vi "HFRR ADV v11.vi"() -> ()   [LabVIEW 2025] (continued)
                    n421 = Bundle By Name(cluster=w701, "average"=w692) -> (w699:cluster{"major":dbl, "minor":dbl, "average":dbl})
                    n422 = Number To Fractional String(number=w692, precision (6)=i16 1) -> (F-format string=w691:string)  [unwired: 2 in]
                    n423 = local write "Minor Axis"(w697) -> ()
                    n424 = local write "Major Axis"(w697) -> ()
                    n425 = Fract/Exp String To Number(string=w691) -> (number=w690:dbl)  [unwired: 3 in, 1 out]
                    n426 = local write "Average"(w690) -> ()
                  }
                }
              }
              frame True {
                w729 = 1000.0 ("y")
                w735 = 0.0 ("default (0 DBL)")
                n427 = Match Pattern(string=w741, regular expression=" \"width_px\":") -> (after substring=w739:string)  [unwired: 1 in, 3 out]
                n428 = Match Pattern(string=w739, regular expression="\"height_px\":") -> (before substring=w737:string, after substring=w736:string)  [unwired: 1 in, 2 out]
                n429 = Fract/Exp String To Number(string=w737, default (0 dbl)=w735) -> (number=w734:dbl)  [unwired: 2 in, 1 out]
                n430 = Fract/Exp String To Number(string=w736, default (0 dbl)=w735) -> (number=w733:dbl)  [unwired: 2 in, 1 out]
                n431 = Multiply(x=w734, y=w732) -> (x*y=w731:dbl)
                n432 = Multiply(x=w733, y=w732) -> (x*y=w730:dbl)
                n433 = Multiply(x=w731, y=w729) -> (x*y=w715:dbl)
                n434 = Multiply(x=w730, y=w729) -> (x*y=w713:dbl)
                n435 = Add(x=w715, y=w713) -> (x+y=w727:dbl)
                n436 = property on="Major Axis" class="DigNum (strict)"("Caption.Text"="Major Axis") -> ()  [unwired: 2 in, 2 out]
                n437 = property on="Minor Axis" class="DigNum (strict)"("Caption.Text"="Minor Axis") -> ()  [unwired: 2 in, 2 out]
                n438 = property on="Average" class="DigNum (strict)"("Caption.Text"="Average") -> ()  [unwired: 2 in, 2 out]
                n439 = Divide(x=w727, y=2.0) -> (x/y=w711:dbl)
                n440 = Bundle By Name(cluster=w728, "major"=w715, "minor"=w713, "average"=w711) -> (w725:cluster{"major":dbl, "minor":dbl, "average":dbl})
                n441 = Number To Fractional String(number=w713, precision (6)=i16 1) -> (F-format string=w720:string)  [unwired: 2 in]
                n442 = Number To Fractional String(number=w711, precision (6)=i16 1) -> (F-format string=w721:string)  [unwired: 2 in]
                n443 = Number To Fractional String(number=w715, precision (6)=i16 1) -> (F-format string=w719:string)  [unwired: 2 in]
                n444 = Fract/Exp String To Number(string=w720) -> (number=w712:dbl)  [unwired: 3 in, 1 out]
                n445 = Fract/Exp String To Number(string=w721) -> (number=w710:dbl)  [unwired: 3 in, 1 out]
                n446 = Fract/Exp String To Number(string=w719) -> (number=w714:dbl)  [unwired: 3 in, 1 out]
                n447 = local write "Major Axis"(w714) -> ()
                n448 = local write "Average"(w710) -> ()
                n449 = local write "Minor Axis"(w712) -> ()
              }
            }
            n450 = case shown="\"Measrument\", Default" w624 {
              tunnel: w627 -> [w654 _]
              tunnel: w626 -> [w653 _]
              tunnel: [w650 w679] -> w625
              tunnel: w623 -> [w652 w679]
              tunnel: w622 -> [w651 _]
              tunnel: w619 -> [w649 _]
              frame "Measrument", Default {
                n451 = stacked-sequence {
                  tunnel: w654 -> [w672 _]
                  tunnel: w653 -> [w670 _]
                  tunnel: w652 -> [w668 _]
                  tunnel: w651 -> [w667 _]
                  tunnel: [w662 _] -> w650
                  tunnel: w649 -> [w655 _]
                  frame #0 {
                    n452 = call "IMAGE ANALYSIS.vi"("Enum"=POST_ANALYSIS_ENUM."SAVE IMAGE", "error in"=w668, "IMAGE FILE PATH"=w667) -> ("error out"=w666:errorcluster)  [unwired: 7 in, 1 out]
                    n453 = call "Stall Data Flow.vim"("value in"=w666, "milliseconds to wait"=u32 1000) -> ("value out"=w657:errorcluster)  [unwired: 1 out]
                    n454 = local read "Test File List :"() -> (w674:string)
                    n455 = call "IMAGE ANALYSIS.vi"("Enum"=POST_ANALYSIS_ENUM."MINIMIZE UI", "error in"=w657) -> ("error out"=w664:errorcluster)  [unwired: 8 in, 1 out]
                    n456 = Bundle By Name(cluster=T21 {"File Name"="", "Test Method"="", "Operator"="", "Fuel Description"="", "Date and time"=""} ("Main Ref"), "Test Method"=w655, "File Name"=w674) -> (w675:T21)
                    n457 = call "Stall Data Flow.vim"("value in"=w664, "milliseconds to wait"=u32 1500) -> ("value out"=w659:errorcluster)  [unwired: 1 out]
                    n458 = call "duf file read.vi"("error in (no error)"=w659, "Main Ref"=w675) -> ("error out"=w673:errorcluster, "Main Ref 2"=w671:T21)  [unwired: 8 in]
                    n459 = call "DETECTION REPORT for manual.vi"("error in (no error)"=w673, "return value 3"=w670, "Image File Path"=w672, "Main Ref"=w671) -> ("error out"=w669:errorcluster)  [unwired: 7 in]
                    n460 = call <vilib>:"Clear Errors.vi"("error in (no error)"=w669) -> ("error out"=w660:errorcluster)  [unwired: 5 in, 1 out]
                    n461 = call "IMAGE ANALYSIS.vi"("Enum"=POST_ANALYSIS_ENUM."MINIMIZE UI", "error in"=w660) -> ("error out"=w662:errorcluster)  [unwired: 8 in, 1 out]
                  }
                  frame #1 {
                    n462 = local write "Main Tab"(T2."HOME" ("Main Tab")) -> ()
                    n463 = local write "Main Dashboard Buttons"(T1."Home" ("Main Dashboard Buttons")) -> ()
                  }
                }
              }
              frame "Calibrate" {
              }
            }
          }
          frame #2 {
            n464 = Not(x=w744) -> (.not. x?=w743:bool)
            n465 = local write "Confirm Measrurement"(w743) -> ()
            n466 = local read "Calibration Tab"() -> (w742:enum32{"Measrument", "Calibrate"})
            n467 = case shown="\"Measrument\", Default" w742 {
              frame "Measrument", Default {
                n468 = local write "Main Tab"(T2."HOME" ("Main Tab")) -> ()
              }
              frame "Calibrate" {
              }
            }
          }
        }
      }
    }
    n469 = local read "Humidity"() -> (w487:bool)
    n470 = local read "Save Change"() -> (w492:bool)
    n471 = local read "Calibrate"() -> (w493:bool)
    n472 = local read "Auto Start Test"() -> (w488:bool)
    n473 = case shown="True" w493 {
      selector: w493 -> [_ w600]
      frame False {
      }
      frame True {
        n474 = Not(x=w600) -> (.not. x?=w599:bool)
        n475 = local write "Calibrate"(w599) -> ()
        n476 = local write "Calibration Tab"(enum32{"Measrument", "Calibrate"}."Calibrate" ("Calibration Tab")) -> ()
      }
    }
    n477 = case shown="True" w492 {
      selector: w492 -> [_ w544]
      frame False {
      }
      frame True {
        n478 = stacked-sequence {
          tunnel: w544 -> [_ _ _ _ w598]
          frame #0 {
            n479 = call "IMAGE ANALYSIS.vi"("Enum"=POST_ANALYSIS_ENUM."HIDE UI") -> ()  [unwired: 9 in, 2 out]
          }
          frame #1 {
            n480 = local read "100x gain"() -> (w546:dbl)
            n481 = local read "10x Gain"() -> (w547:dbl)
            n482 = local read "5x Gain"() -> (w548:dbl)
            n483 = Number To Fractional String(number=w547, width (-)=i16 4, precision (6)=i16 7) -> (F-format string=w569:string)  [unwired: 1 in]
            n484 = Number To Fractional String(number=0.0, width (-)=i16 4, precision (6)=i16 7) -> (F-format string=w564:string)  [unwired: 1 in]
            n485 = Number To Fractional String(number=w546, width (-)=i16 4, precision (6)=i16 7) -> (F-format string=w552:string)  [unwired: 1 in]
            n486 = Number To Fractional String(number=w548, width (-)=i16 10 ("precision (6)"), precision (6)=i16 7) -> (F-format string=w578:string)  [unwired: 1 in]
            n487 = Concatenate Strings("[CH1]" ("string"), w578, " - 5x Gain" ("string"), "\r") -> (w568:string)
            n488 = Concatenate Strings("[CH2]" ("string"), w569, " - 10x Gain" ("string"), "\r") -> (w567:string)
            n489 = Concatenate Strings("[CH3]" ("string"), w564, " - 20x Gain" ("string"), "\r") -> (w558:string)
            n490 = Concatenate Strings("[CH4]" ("string"), w552, " - 100x Gain" ("string"), "\r") -> (w551:string)
            n491 = String To Path(string="C:\\LAB-IQ\\Image Calibrate v01.dcf") -> (path=w581:path)
            n492 = Concatenate Strings(w568, w567, w558, w551) -> (w566:string)
            n493 = call <vilib>:"Write Characters To File.vi"("append to file? (new file:F)"=FALSE, "character string"=w566, "file path (dialog if empty)"=w581) -> ()  [unwired: 2 in, 1 out]
          }
          frame #2 {
            n494 = String To Path(string="C:\\LAB-IQ\\Image Calibrate v01.dcf") -> (path=w584:path)
            n495 = Open/Create/Replace File ("Open File")(file path (use dialog)=w584) -> (refnum out=w585:refnum<file>)  [unwired: 5 in, 2 out]
            n496 = for {
              N: 4 -> [_]
              tunnel: w585 -> [w591]
              i -> [w587]
              n497 = Read from Text File ("Read File")(file (use dialog)=w591) -> (text=w592:string)  [unwired: 3 in, 3 out]
              n498 = String Subset(string=w592, offset (0)=6, length (rest)=10 ("length (rest)")) -> (substring=w588:string)
              n499 = Fract/Exp String To Number(string=w588) -> (number=w586:dbl)  [unwired: 3 in, 1 out]
              n500 = case shown="3" w587 {
                tunnel: w586 -> [w593 w594 _ w595 _]
                frame 0 {
                  n501 = local write "5x Gain"(w593) -> ()
                }
                frame 1 {
                  n502 = local write "10x Gain"(w594) -> ()
                }
                frame 2 {
                }
                frame 3 {
                  n503 = local write "100x gain"(w595) -> ()
                }
                frame 4, Default {
                }
              }
            }
          }
          frame #3 {
            n504 = call "IMAGE ANALYSIS.vi"("Enum"=POST_ANALYSIS_ENUM."SHOW UI") -> ()  [unwired: 9 in, 2 out]
          }
          frame #4 {
            n505 = Not(x=w598) -> (.not. x?=w597:bool)
            n506 = local write "Save Change"(w597) -> ()
          }
        }
      }
    }
    n507 = case shown="False" w488 {
      tunnel: w487 -> [w514 _]
      frame False {
        n508 = case shown="True" w514 {
          frame False {
          }
          frame True {
            n509 = local read "Set Humidity:"() -> (w518:dbl)
            n510 = local read "Set Humidity:"() -> (w521:dbl)
            n511 = local read "Humidity ( %RH )"() -> (w522:dbl)
            n512 = Subtract(x=w518, y=2.0) -> (x-y=w516:dbl)
            n513 = Add(x=w521, y=2.0) -> (x+y=w517:dbl)
            n514 = In Range and Coerce(upper limit=w517, x=w522, lower limit=w516) -> (In Range?=w515:bool)  [unwired: 1 out]
            n515 = case shown="True" w515 {
              frame False {
              }
              frame True {
                n516 = case shown="False" "Manual Humididty Reached" {
                  selector: "Manual Humididty Reached" -> [_ w525]
                  frame False {
                  }
                  frame True {
                    n517 = Not(x=w525) -> (.not. x?=w524:bool)
                    n518 = local write "Manual Humididty Reached"(w524) -> ()
                    n519 = local read "EVENT LOG"() -> (w527:string)
                    n520 = call "Event Log.vi"("Content"="Target Humidity reached", "EVENT LOG"=w527) -> ("EVENT LOG"=w526:string)  [unwired: 8 in, 1 out]
                    n521 = local write "EVENT LOG"(w526) -> ()
                  }
                }
              }
            }
          }
        }
      }
      frame True {
        n522 = local write "Manual Humididty Reached"(TRUE ("Manual Humididty Reached")) -> ()
      }
    }
    n523 = local read "Cap Live Image"() -> (w508:bool)
    n524 = local read "SCAR MEASURMENT"() -> (w511:enum32{"Auto Scar", "Manual Scar"})
    n525 = Wait (ms)(milliseconds to wait=u32 250) -> ()  [unwired: 1 out]
    n526 = Equal?(x=w511, y=enum32{"Auto Scar", "Manual Scar"}."Manual Scar" ("SCAR MEASURMENT")) -> (x = y?=w509:bool)
    n527 = And(x=w509, y=w508) -> (x .and. y?=w507:bool)
    n528 = case shown="True" w507 {
      selector: w507 -> [_ w823]
      frame False {
      }
      frame True {
        n529 = stacked-sequence {
          tunnel: [_ _ _ w838 _] -> _
          tunnel: w823 -> [_ _ _ _ w844]
          frame #0 {
            w824 = 0.0
            n530 = local write "Major Axis"(w824) -> ()
            n531 = local write "Minor Axis"(w824) -> ()
            n532 = local write "Average"(w824) -> ()
          }
          frame #1 {
            n533 = call "CAMERA LIVE FEED FGV.vi"("Enum - Menu"=CAMERA_LIVE_FEED_ENUM."CAMERA MINIMIZE") -> ()  [unwired: 9 in, 2 out]
          }
          frame #2 {
            n534 = local read "FILE 3"() -> (w832:string)
            n535 = call <vilib>:"Trim Whitespace.vi"("string"="C:\\LAB-IQ\\images\\") -> ("trimmed string"=w834:string)  [unwired: 1 in]
            n536 = String To Path(string=w834) -> (path=w833:path)
            n537 = Concatenate Strings(w832, ".png" ("string")) -> (w831:string)
            n538 = Build Path(base path=w833, name or relative path=w831) -> (appended path=w829:path)
            n539 = Path To String(path=w829) -> (string=w828:string)
            n540 = call "CAMERA LIVE FEED FGV.vi"("Enum - Menu"=CAMERA_LIVE_FEED_ENUM."CAMERA SAVE", "Image Path"=w828) -> ("error out"=w826:errorcluster)  [unwired: 8 in, 1 out]
            n541 = case shown="No Error" w826 {
              frame No Error {
                n542 = One Button Dialog(message="Image saved successfully") -> ()  [unwired: 1 in, 1 out]
              }
              frame Error {
              }
            }
          }
          frame #3 {
            n543 = call "LIST FILE NAMES.vi"() -> ("error out"=w840:errorcluster, "filenames"=w837:string[])  [unwired: 10 in]
            n544 = call "IMAGE ANALYSIS.vi"("Enum"=POST_ANALYSIS_ENUM."SHOW UI", "error in"=w840) -> ("error out"=w838:errorcluster)  [unwired: 8 in, 1 out]
            n545 = property on="Test File List :" class="CmbBox"("Strings[]"=w837) -> ()  [unwired: 2 in, 2 out]
          }
          frame #4 {
            (unwired) T22."Report" ("Main Dashboard Buttons")
            n546 = Not(x=w844) -> (.not. x?=w843:bool)
            n547 = local write "Zoom Factore"(0.0 ("Zoom Factore")) -> ()
            n548 = local write "Cap Live Image"(w843) -> ()
            n549 = local write "Main Tab"(T2."Adv Scar Report" ("Main Tab")) -> ()
            n550 = property on="Cap Live Image" class="Bool (strict)"("BoolText.Text"="Capture Image" ("Boolean Text.Text")) -> ()  [unwired: 2 in, 2 out]
            n551 = local write "Main Dashboard Buttons"(T1."Report" ("Main Dashboard Buttons")) -> ()
          }
        }
      }
    }
    n552 = local read "change Gain"() -> (w491:bool)
    n553 = local read "Back Square"() -> (w490:bool)
    n554 = case shown="True" w491 {
      selector: w491 -> [_ w535]
      frame False {
      }
      frame True {
        n555 = stacked-sequence {
          tunnel: w535 -> [_ w543]
          frame #0 {
            n556 = local read "Actual (µm)"() -> (w539:dbl)
            n557 = local read "Pixel Value"() -> (w538:dbl)
            n558 = local read "Magnification :"() -> (w537:string)
            n559 = Divide(x=w539, y=w538) -> (x/y=w536:dbl)
            n560 = case shown="\"10x\"" w537 {
              tunnel: w536 -> [w540 w541]
              frame "10x" {
                n561 = local write "10x Gain"(w540) -> ()
              }
              frame "5x", Default {
                n562 = local write "5x Gain"(w541) -> ()
              }
            }
          }
          frame #1 {
            n563 = Not(x=w543) -> (.not. x?=w542:bool)
            n564 = local write "change Gain"(w542) -> ()
          }
        }
      }
    }
    n565 = case shown="True" w490 {
      selector: w490 -> [_ w533]
      frame False {
      }
      frame True {
        n566 = Not(x=w533) -> (.not. x?=w532:bool)
        n567 = local write "Back Square"(w532) -> ()
        n568 = local write "Calibration Tab"(enum32{"Measrument", "Calibrate"}."Measrument" ("Calibration Tab")) -> ()
      }
    }
    n569 = local read "Rectangle Tool"() -> (w502:bool)
    n570 = local read "Clear ROI Tool"() -> (w501:bool)
    n571 = local read "Open Image"() -> (w506:bool)
    n572 = local read "line tool"() -> (w503:bool)
    n573 = local read "OUT"() -> (w504:bool)
    n574 = local read "In"() -> (w505:bool)
    n575 = case shown="True" w506 {
      selector: w506 -> [_ w811]
      tunnel: [w807 w813] -> _
      tunnel: w496 -> [w807 w812]
      frame False {
      }
      frame True {
        n576 = Not(x=w811) -> (.not. x?=w810:bool)
        n577 = local write "Open Image"(w810) -> ()
        n578 = call "IMAGE ANALYSIS.vi"("Enum"=POST_ANALYSIS_ENUM."HIDE UI", "error in"=w812) -> ("error out"=w820:errorcluster)  [unwired: 8 in, 1 out]
        n579 = call "File Dialog"("start path"=path "C:/LAB-IQ/images", "error in"=w820) -> ("selected path"=w809:path, "error out"=w818:errorcluster)  [unwired: 10 in, 2 out]
        "Image path  2" <- w809
        n580 = call <vilib>:"Clear Errors.vi"("error in (no error)"=w818) -> ("error out"=w817:errorcluster)  [unwired: 5 in, 1 out]
        n581 = call "IMAGE ANALYSIS.vi"("Enum"=POST_ANALYSIS_ENUM."OPEN FILE", "error in"=w817, "File Path"=w809) -> ("error out"=w816:errorcluster)  [unwired: 7 in, 1 out]
        n582 = call <vilib>:"Clear Errors.vi"("error in (no error)"=w816) -> ("error out"=w815:errorcluster)  [unwired: 5 in, 1 out]
        n583 = call "IMAGE ANALYSIS.vi"("Enum"=POST_ANALYSIS_ENUM."SHOW UI", "error in"=w815) -> ("error out"=w813:errorcluster)  [unwired: 8 in, 1 out]
        n584 = local write "Zoom Factore"(100.0 ("Zoom Factore")) -> ()
      }
    }
    n585 = case shown="True" w504 {
      selector: w504 -> [_ w792]
      tunnel: w496 -> [w789 w797]
      tunnel: [w789 w791] -> _
      frame False {
      }
      frame True {
        n586 = Not(x=w792) -> (.not. x?=w790:bool)
        n587 = local read "Zoom Factore"() -> (w795:dbl)
        n588 = local write "OUT"(w790) -> ()
        n589 = call "IMAGE ANALYSIS.vi"("Enum"=POST_ANALYSIS_ENUM."ZOOM OUT", "error in"=w797) -> ("error out"=w791:errorcluster)  [unwired: 8 in, 1 out]
        n590 = Divide(x=w795, y=1.2) -> (x/y=w793:dbl)
        n591 = local write "Zoom Factore"(w793) -> ()
      }
    }
    n592 = case shown="True" w505 {
      selector: w505 -> [_ w801]
      tunnel: w496 -> [w798 w806]
      tunnel: [w798 w799] -> _
      frame False {
      }
      frame True {
        n593 = Not(x=w801) -> (.not. x?=w800:bool)
        n594 = local read "Zoom Factore"() -> (w804:dbl)
        n595 = local write "In"(w800) -> ()
        n596 = call "IMAGE ANALYSIS.vi"("Enum"=POST_ANALYSIS_ENUM."ZOOM IN", "error in"=w806) -> ("error out"=w799:errorcluster)  [unwired: 8 in, 1 out]
        n597 = Multiply(x=w804, y=1.2) -> (x*y=w802:dbl)
        n598 = local write "Zoom Factore"(w802) -> ()
      }
    }
    n599 = case shown="True" w501 {
      selector: w501 -> [_ w773]
      tunnel: w496 -> [w771 w775]
      tunnel: [w771 w774] -> _
      frame False {
      }
      frame True {
        n600 = Not(x=w773) -> (.not. x?=w772:bool)
        n601 = local write "Clear ROI Tool"(w772) -> ()
        n602 = call "IMAGE ANALYSIS.vi"("Enum"=POST_ANALYSIS_ENUM."CLEAR ROI", "error in"=w775) -> ("error out"=w774:errorcluster)  [unwired: 8 in, 1 out]
      }
    }
    n603 = case shown="True" w503 {
      selector: w503 -> [_ w785]
      tunnel: w496 -> [w783 w788]
      tunnel: [w783 w786] -> _
      frame False {
      }
      frame True {
        n604 = Not(x=w785) -> (.not. x?=w784:bool)
        n605 = local write "line tool"(w784) -> ()
        n606 = call "IMAGE ANALYSIS.vi"("Enum"=POST_ANALYSIS_ENUM."DRAW LINE", "error in"=w788) -> ("error out"=w786:errorcluster)  [unwired: 8 in, 1 out]
      }
    }
    n607 = case shown="True" w502 {
      selector: w502 -> [_ w779]
      tunnel: w496 -> [w777 w781]
      tunnel: [w777 w780] -> _
      frame False {
      }
      frame True {
        n608 = Not(x=w779) -> (.not. x?=w778:bool)
        n609 = local write "Rectangle Tool"(w778) -> ()
        n610 = call "IMAGE ANALYSIS.vi"("Enum"=POST_ANALYSIS_ENUM."DRAW REC", "error in"=w781) -> ("error out"=w780:errorcluster)  [unwired: 8 in, 1 out]
      }
    }
    n611 = local read "SCAR MEASURMENT"() -> (w489:enum32{"Auto Scar", "Manual Scar"})
    n612 = local read "Fit to Screen Tool"() -> (w498:bool)
    n613 = local read "Resize Tool"() -> (w497:bool)
    n614 = case shown="\"Manual Scar\", Default" w489 {
      frame "Auto Scar" {
        n615 = property on="Cap Live Image" class="Bool (strict)"("BoolText.Text"="Report" ("Boolean Text.Text")) -> ()  [unwired: 2 in, 2 out]
      }
      frame "Manual Scar", Default {
        n616 = property on="Cap Live Image" class="Bool (strict)"("BoolText.Text"="Save Image" ("Boolean Text.Text")) -> ()  [unwired: 2 in, 2 out]
      }
    }
    n617 = local read "ROI Color Tool"() -> (w499:bool)
    n618 = local read "Pan Tool"() -> (w500:bool)
    n619 = case shown="True" w500 {
      selector: w500 -> [_ w767]
      tunnel: w496 -> [w765 w769]
      tunnel: [w765 w768] -> _
      frame False {
      }
      frame True {
        n620 = Not(x=w767) -> (.not. x?=w766:bool)
        n621 = call "IMAGE ANALYSIS.vi"("Enum"=POST_ANALYSIS_ENUM."PAN", "error in"=w769) -> ("error out"=w768:errorcluster)  [unwired: 8 in, 1 out]
        n622 = local write "Pan Tool"(w766) -> ()
      }
    }
    n623 = case shown="True" w497 {
      selector: w497 -> [_ w751]
      tunnel: w496 -> [w746 w748]
      tunnel: [w746 w747] -> _
      frame False {
      }
      frame True {
        n624 = Not(x=w751) -> (.not. x?=w750:bool)
        n625 = local write "Resize Tool"(w750) -> ()
        n626 = call "IMAGE ANALYSIS.vi"("Enum"=POST_ANALYSIS_ENUM."RESIZE MODE", "error in"=w748) -> ("error out"=w747:errorcluster)  [unwired: 8 in, 1 out]
      }
    }
    n627 = case shown="True" w498 {
      selector: w498 -> [_ w756]
      tunnel: [w752 w757] -> _
      tunnel: w496 -> [w752 w755]
      frame False {
      }
      frame True {
        n628 = Not(x=w756) -> (.not. x?=w754:bool)
        n629 = local write "Zoom Factore"(100.0 ("Zoom Factore")) -> ()
        n630 = local write "Fit to Screen Tool"(w754) -> ()
        n631 = call "IMAGE ANALYSIS.vi"("Enum"=POST_ANALYSIS_ENUM."FIT", "error in"=w755) -> ("error out"=w757:errorcluster)  [unwired: 8 in, 1 out]
      }
    }
    n632 = case shown="True" w499 {
      selector: w499 -> [_ w762]
      tunnel: [w759 w763] -> _
      tunnel: w496 -> [w759 w760]
      frame False {
      }
      frame True {
        n633 = Not(x=w762) -> (.not. x?=w761:bool)
        n634 = local write "ROI Color Tool"(w761) -> ()
        n635 = call "IMAGE ANALYSIS.vi"("Enum"=POST_ANALYSIS_ENUM."SET ROI COLOR", "error in"=w760) -> ("error out"=w763:errorcluster)  [unwired: 8 in, 1 out]
      }
    }
    n636 = local read "Quit"() -> (w513:bool)
  }
  n637 = local write "USERNAME"(w28) -> ()
  n638 = local write "Main Tab"(T2."HOME" ("Main Tab")) -> ()
  n639 = local write "USER ID"(w28) -> ()
  n640 = property on="Auto Scar Check  2" class="Clust (strict)"("Visible"=w9) -> (error out=w13:errorcluster)  [unwired: 2 in, 1 out]
  n641 = property on="Quit" class="Bool (strict)"("Value"=FALSE ("Quit")) -> (error out=w30:errorcluster)  [unwired: 2 in, 1 out]
  n642 = while {
    stop <- w847 stop-if-true
    n643 = local read "Image Path"() -> (w850:path)
    n644 = local read "Print 3"() -> (w853:bool)
    n645 = Equal?(x=w850, y=path "") -> (x = y?=w849:bool)
    n646 = Not(x=w849) -> (.not. x?=w848:bool)
    n647 = property on="Print 3" class="Bool (strict)"("Visible"=w848) -> ()  [unwired: 2 in, 2 out]
    n648 = case shown="True" w853 {
      frame False {
        n649 = local write "Rd"(TRUE ("Boolean 7")) -> ()
      }
      frame True {
        n650 = flat-sequence {
          tunnel: [w893] -> w861
          tunnel: [w880] -> w859
          tunnel: [w890] -> w855
          tunnel: w861 -> [w902]
          tunnel: [w902] -> w860
          tunnel: w859 -> [w901]
          tunnel: [w901] -> w858
          tunnel: [w899] -> w857
          tunnel: [w898] -> w856
          tunnel: w855 -> [w898]
          tunnel: w860 -> [w904]
          tunnel: w858 -> [w905]
          tunnel: w857 -> [_]
          tunnel: w856 -> [w903]
          frame #0 {
            n651 = case shown="True" "Rd" {
              frame False {
              }
              frame True {
                n652 = while {
                  tunnel: "abcdefABCDEF" ("string 2") -> [w872]
                  shift-right: [w870] -> w864
                  shift-left: "" -> [w869]
                  i -> [w879]
                  stop <- w878 stop-if-true
                  n653 = Random Number (0-1)() -> (number: 0 to 1=w873:dbl)
                  n654 = Multiply(x=w873, y=62.0) -> (x*y=w875:dbl)
                  n655 = Decrement(x="Length 2") -> (x-1=w868:i16)
                  n656 = To Word Integer(number=w875) -> (16bit integer=w876:i16)
                  n657 = String Subset(string=w872, offset (0)=w876, length (rest)=1 ("length (rest)")) -> (substring=w871:string)
                  n658 = Greater Or Equal?(x=w879, y=w868) -> (x >= y?=w878:bool)
                  n659 = Concatenate Strings(w871, w869) -> (w870:string)
                }
                "String 10" <- w864
                n660 = local write "Rd"(FALSE ("Boolean 7")) -> ()
              }
            }
          }
          frame #1 {
            w891 = "_resized.jpg" ("command line")
            (unwired) ".jpg -resize 320x240 " ("string")
            (unwired) "Choose an Image File" ("prompt")
            # "-resize 1798x425"
            n661 = local read "Image Path"() -> (w885:path)
            n662 = Strip Path(path=w885) -> (stripped path=w880:path, name=w881:string)
            n663 = Match Pattern(string=w881, regular expression=".jpg") -> (before substring=→"before substring 2":string, after substring=→"after substring":string)  [unwired: 1 in, 2 out]
            n664 = Match Pattern(string=w881, regular expression="\\") -> (before substring=w887:string)  [unwired: 1 in, 3 out]
            n665 = Match Pattern(string=w887, regular expression=".jpg") -> (before substring=w886:string)  [unwired: 1 in, 3 out]
            n666 = Concatenate Strings("cmd /c convert " ("string"), w886, ".jpg -resize 320x240  " ("command line"), w886, w891) -> (w894:string)
            n667 = call <vilib>:"System Exec.vi"("run minimized? (F)"=TRUE, "wait until completion? (T)"=TRUE, "working directory"=w880, "command line"=w894) -> ("error out"=w893:errorcluster)  [unwired: 4 in, 3 out]
            "error out 2" <- w893
            n668 = Concatenate Strings(w886, w891) -> (w890:string)
          }
          frame #2 {
            n669 = Wait (ms)(milliseconds to wait=u32 2000 ("millisecond timer value")) -> (millisecond timer value=w899:u32)
          }
          frame #3 {
            n670 = case shown="No Error" w904 {
              tunnel: w905 -> [w908 _]
              tunnel: w903 -> [w906 _]
              frame No Error {
                (unwired) ".jpg" ("string")
                n671 = Path To String(path=w908) -> (string=w912:string)
                n672 = Concatenate Strings(w912, "\\" ("string"), w906) -> (w911:string)
                n673 = String To Path(string=w911) -> (path=w910:path)
                n674 = call <vilib>:"Read JPEG File.vi"("path to JPEG file"=w910) -> ("image data"=w914:T14)  [unwired: 8 in, 2 out]
                "image data" <- w914
                n675 = local write "Print 3"(FALSE ("Print 2")) -> ()
                n676 = call <vilib>:"Draw Flattened Pixmap.vi"("image data"=w914) -> ("new picture"=→"new picture":picture)  [unwired: 8 in]
              }
              frame Error {
              }
            }
          }
        }
      }
    }
    n677 = Wait (ms)(milliseconds to wait=u32 20 ("millisecond timer value")) -> ()  [unwired: 1 out]
    n678 = local read "Quit"() -> (w847:bool)
  }
  n679 = property on="Service Password Log" class="Str"("Visible"=w9) -> ()  [unwired: 2 in, 2 out]
  n680 = property on="Password 3" class="Clust (strict)"("Visible"=w9) -> ()  [unwired: 2 in, 2 out]
  n681 = while {
    tunnel: w30 -> [_]
    tunnel: w13 -> [_]
    stop <- w945 stop-if-true
    # "New Adv Logics"
    n682 = local read "Main Tab"() -> (w943:T2)
    n683 = local read "Sign In"() -> (w942:bool)
    n684 = local read "Main Tab"() -> (w924:T2)
    n685 = case shown="\"Mooha\"" w924 {
      frame "HOME", Default {
        n686 = local read "LIVE FEED MIN TEMP"() -> (w1072:bool)
        n687 = local write "LIVE FEED MAX TEMP"(TRUE ("LIVE FEED MAX TEMP")) -> ()
        n688 = local read "CAMERA ROI MIN TEMP"() -> (w1070:bool)
        n689 = case shown="True" w1072 {
          selector: w1072 -> [_ w1079]
          frame False {
          }
          frame True {
            n690 = Not(x=w1079) -> (.not. x?=w1078:bool)
            n691 = local write "LIVE FEED MIN TEMP"(w1078) -> ()
            n692 = call "CAMERA LIVE FEED FGV.vi"("Enum - Menu"=CAMERA_LIVE_FEED_ENUM."CAMERA MINIMIZE") -> ()  [unwired: 9 in, 2 out]
          }
        }
        n693 = case shown="True" w1070 {
          selector: w1070 -> [_ w1076]
          frame False {
          }
          frame True {
            n694 = Not(x=w1076) -> (.not. x?=w1075:bool)
            n695 = local write "CAMERA ROI MIN TEMP"(w1075) -> ()
            n696 = call "IMAGE ANALYSIS.vi"("Enum"=POST_ANALYSIS_ENUM."MINIMIZE UI") -> ()  [unwired: 9 in, 2 out]
          }
        }
        n697 = local write "CAMERA ROI MAX TEMP"(TRUE ("CAMERA ROI MAX TEMP")) -> ()
      }
      frame "Test Setup" {
        n698 = local read "LIVE FEED MIN TEMP"() -> (w1082:bool)
        n699 = local read "CAMERA ROI MIN TEMP"() -> (w1080:bool)
        n700 = local write "LIVE FEED MAX TEMP"(TRUE ("LIVE FEED MAX TEMP")) -> ()
        n701 = case shown="True" w1082 {
          selector: w1082 -> [_ w1089]
          frame False {
          }
          frame True {
            n702 = Not(x=w1089) -> (.not. x?=w1088:bool)
            n703 = local write "LIVE FEED MIN TEMP"(w1088) -> ()
            n704 = call "CAMERA LIVE FEED FGV.vi"("Enum - Menu"=CAMERA_LIVE_FEED_ENUM."CAMERA MINIMIZE") -> ()  [unwired: 9 in, 2 out]
          }
        }
        n705 = case shown="True" w1080 {
          selector: w1080 -> [_ w1086]
          frame False {
          }
          frame True {
            n706 = Not(x=w1086) -> (.not. x?=w1085:bool)
            n707 = local write "CAMERA ROI MIN TEMP"(w1085) -> ()
            n708 = call "IMAGE ANALYSIS.vi"("Enum"=POST_ANALYSIS_ENUM."MINIMIZE UI") -> ()  [unwired: 9 in, 2 out]
          }
        }
        n709 = local write "CAMERA ROI MAX TEMP"(TRUE ("CAMERA ROI MAX TEMP")) -> ()
      }
      frame "Acquire" {
        n710 = local read "LIVE FEED MIN TEMP"() -> (w1092:bool)
        n711 = local write "LIVE FEED MAX TEMP"(TRUE ("LIVE FEED MAX TEMP")) -> ()
        n712 = local read "CAMERA ROI MIN TEMP"() -> (w1090:bool)
        n713 = case shown="True" w1092 {
          selector: w1092 -> [_ w1099]
          frame False {
          }
          frame True {
            n714 = Not(x=w1099) -> (.not. x?=w1098:bool)
            n715 = local write "LIVE FEED MIN TEMP"(w1098) -> ()
            n716 = call "CAMERA LIVE FEED FGV.vi"("Enum - Menu"=CAMERA_LIVE_FEED_ENUM."CAMERA MINIMIZE") -> ()  [unwired: 9 in, 2 out]
          }
        }
        n717 = case shown="True" w1090 {
          selector: w1090 -> [_ w1096]
          frame False {
          }
          frame True {
            n718 = Not(x=w1096) -> (.not. x?=w1095:bool)
            n719 = local write "CAMERA ROI MIN TEMP"(w1095) -> ()
            n720 = call "IMAGE ANALYSIS.vi"("Enum"=POST_ANALYSIS_ENUM."MINIMIZE UI") -> ()  [unwired: 9 in, 2 out]
          }
        }
        n721 = local write "CAMERA ROI MAX TEMP"(TRUE ("CAMERA ROI MAX TEMP")) -> ()
      }
      frame "Adv Scar" {
        n722 = local read "CAMERA ROI MIN TEMP"() -> (w1100:bool)
        n723 = case shown="True" "LIVE FEED MAX TEMP" {
          selector: "LIVE FEED MAX TEMP" -> [_ w1119]
          frame False {
          }
          frame True {
            n724 = Not(x=w1119) -> (.not. x?=w1118:bool)
            n725 = local write "LIVE FEED MAX TEMP"(w1118) -> ()
            n726 = call "CAMERA LIVE FEED FGV.vi"("Enum - Menu"=CAMERA_LIVE_FEED_ENUM."CAMERA RESTORE") -> ("error out"=w1109:errorcluster)  [unwired: 9 in, 1 out]
            n727 = Type Cast(type=30, x=0) -> (*(type *) &x=w1113:i32)
            n728 = Add(x=w1113, y=48) -> (x+y=w1114:i32)
            n729 = call "CAMERA LIVE FEED FGV.vi"("Enum - Menu"=CAMERA_LIVE_FEED_ENUM."CAMERA MODE SET", "error in (no error)"=w1109, "CAMERA MODE"=w1114) -> ("error out"=w1107:errorcluster)  [unwired: 7 in, 1 out]
            n730 = call "LIST FILE NAMES.vi"("error in (no error)"=w1107) -> ("error out"=w1115:errorcluster, "filenames"=w1116:string[])  [unwired: 9 in]
            n731 = property on="FILE 3" class="CmbBox"(error in=w1115, "Strings[]"=w1116) -> ()  [unwired: 1 in, 2 out]
          }
        }
        n732 = case shown="True" w1100 {
          selector: w1100 -> [_ w1106]
          frame False {
          }
          frame True {
            n733 = Not(x=w1106) -> (.not. x?=w1105:bool)
            n734 = local write "CAMERA ROI MIN TEMP"(w1105) -> ()
            n735 = call "IMAGE ANALYSIS.vi"("Enum"=POST_ANALYSIS_ENUM."MINIMIZE UI") -> ()  [unwired: 9 in, 2 out]
          }
        }
        n736 = local write "CAMERA ROI MAX TEMP"(TRUE ("CAMERA ROI MAX TEMP")) -> ()
        "LIVE FEED MIN TEMP" <- TRUE ("LIVE FEED MIN TEMP")
      }
      frame "Adv Scar Report" {
        n737 = local read "CAMERA ROI MAX TEMP"() -> (w1120:bool)
        n738 = local read "LIVE FEED MIN TEMP"() -> (w1122:bool)
        n739 = local write "LIVE FEED MAX TEMP"(TRUE ("LIVE FEED MAX TEMP")) -> ()
        n740 = case shown="True" w1122 {
          selector: w1122 -> [_ w1131]
          frame False {
          }
          frame True {
            n741 = Not(x=w1131) -> (.not. x?=w1130:bool)
            n742 = local write "LIVE FEED MIN TEMP"(w1130) -> ()
            n743 = call "CAMERA LIVE FEED FGV.vi"("Enum - Menu"=CAMERA_LIVE_FEED_ENUM."CAMERA MINIMIZE") -> ()  [unwired: 9 in, 2 out]
          }
        }
        n744 = case shown="True" w1120 {
          selector: w1120 -> [_ w1128]
          frame False {
          }
          frame True {
            n745 = Not(x=w1128) -> (.not. x?=w1126:bool)
            n746 = local write "CAMERA ROI MAX TEMP"(w1126) -> ()
            n747 = call "IMAGE ANALYSIS.vi"("Enum"=POST_ANALYSIS_ENUM."SHOW UI") -> ("error out"=w1125:errorcluster)  [unwired: 9 in, 1 out]
            n748 = call "LIST FILE NAMES.vi"("error in (no error)"=w1125) -> ("filenames"=w1124:string[])  [unwired: 9 in, 1 out]
            n749 = property on="Test File List :" class="CmbBox"("Strings[]"=w1124) -> ()  [unwired: 2 in, 2 out]
          }
        }
        n750 = local write "CAMERA ROI MIN TEMP"(TRUE ("CAMERA ROI MIN TEMP")) -> ()
      }
      frame "Compare Files" {
        n751 = local read "LIVE FEED MIN TEMP"() -> (w1134:bool)
        n752 = local write "LIVE FEED MAX TEMP"(TRUE ("LIVE FEED MAX TEMP")) -> ()
        n753 = local read "CAMERA ROI MIN TEMP"() -> (w1132:bool)
        n754 = case shown="True" w1134 {
          selector: w1134 -> [_ w1141]
          frame False {
          }
          frame True {
            n755 = Not(x=w1141) -> (.not. x?=w1140:bool)
            n756 = local write "LIVE FEED MIN TEMP"(w1140) -> ()
            n757 = call "CAMERA LIVE FEED FGV.vi"("Enum - Menu"=CAMERA_LIVE_FEED_ENUM."CAMERA MINIMIZE") -> ()  [unwired: 9 in, 2 out]
          }
        }
        n758 = case shown="True" w1132 {
          selector: w1132 -> [_ w1138]
          frame False {
          }
          frame True {
            n759 = Not(x=w1138) -> (.not. x?=w1137:bool)
            n760 = local write "CAMERA ROI MIN TEMP"(w1137) -> ()
            n761 = call "IMAGE ANALYSIS.vi"("Enum"=POST_ANALYSIS_ENUM."MINIMIZE UI") -> ()  [unwired: 9 in, 2 out]
          }
        }
        n762 = local write "CAMERA ROI MAX TEMP"(TRUE ("CAMERA ROI MAX TEMP")) -> ()
      }
      frame "About" {
        n763 = local read "LIVE FEED MIN TEMP"() -> (w1144:bool)
        n764 = local write "LIVE FEED MAX TEMP"(TRUE ("LIVE FEED MAX TEMP")) -> ()
        n765 = local read "CAMERA ROI MIN TEMP"() -> (w1143:bool)
        n766 = case shown="True" w1144 {
          selector: w1144 -> [_ w1151]
          frame False {
          }
          frame True {
            n767 = Not(x=w1151) -> (.not. x?=w1150:bool)
            n768 = local write "LIVE FEED MIN TEMP"(w1150) -> ()
            n769 = call "CAMERA LIVE FEED FGV.vi"("Enum - Menu"=CAMERA_LIVE_FEED_ENUM."CAMERA MINIMIZE") -> ()  [unwired: 9 in, 2 out]
          }
        }
        n770 = case shown="True" w1143 {
          selector: w1143 -> [_ w1148]
          frame False {
          }
          frame True {
            n771 = Not(x=w1148) -> (.not. x?=w1147:bool)
            n772 = local write "CAMERA ROI MIN TEMP"(w1147) -> ()
            n773 = call "IMAGE ANALYSIS.vi"("Enum"=POST_ANALYSIS_ENUM."MINIMIZE UI") -> ()  [unwired: 9 in, 2 out]
          }
        }
        n774 = local write "CAMERA ROI MAX TEMP"(TRUE ("CAMERA ROI MIN TEMP")) -> ()
      }
      frame "Advance" {
        n775 = local read "LIVE FEED MIN TEMP"() -> (w1154:bool)
        n776 = local write "LIVE FEED MAX TEMP"(TRUE ("LIVE FEED MAX TEMP")) -> ()
        n777 = local read "CAMERA ROI MIN TEMP"() -> (w1152:bool)
        n778 = case shown="True" w1154 {
          selector: w1154 -> [_ w1161]
          frame False {
          }
          frame True {
            n779 = Not(x=w1161) -> (.not. x?=w1160:bool)
            n780 = local write "LIVE FEED MIN TEMP"(w1160) -> ()
            n781 = call "CAMERA LIVE FEED FGV.vi"("Enum - Menu"=CAMERA_LIVE_FEED_ENUM."CAMERA MINIMIZE") -> ()  [unwired: 9 in, 2 out]
          }
        }
        n782 = local write "CAMERA ROI MAX TEMP"(TRUE ("CAMERA ROI MAX TEMP")) -> ()
        n783 = case shown="True" w1152 {
          selector: w1152 -> [_ w1158]
          frame False {
          }
          frame True {
            n784 = Not(x=w1158) -> (.not. x?=w1157:bool)
            n785 = local write "CAMERA ROI MIN TEMP"(w1157) -> ()
            n786 = call "IMAGE ANALYSIS.vi"("Enum"=POST_ANALYSIS_ENUM."MINIMIZE UI") -> ()  [unwired: 9 in, 2 out]
          }
        }
      }
      frame "Mooha" {
        n787 = local read "LIVE FEED MIN TEMP"() -> (w1164:bool)
        n788 = local write "LIVE FEED MAX TEMP"(TRUE ("LIVE FEED MAX TEMP")) -> ()
        n789 = local read "CAMERA ROI MIN TEMP"() -> (w1162:bool)
        n790 = case shown="True" w1164 {
          selector: w1164 -> [_ w1171]
          frame False {
          }
          frame True {
            n791 = Not(x=w1171) -> (.not. x?=w1170:bool)
            n792 = local write "LIVE FEED MIN TEMP"(w1170) -> ()
            n793 = call "CAMERA LIVE FEED FGV.vi"("Enum - Menu"=CAMERA_LIVE_FEED_ENUM."CAMERA MINIMIZE") -> ()  [unwired: 9 in, 2 out]
          }
        }
        n794 = local write "CAMERA ROI MAX TEMP"(TRUE ("CAMERA ROI MAX TEMP")) -> ()
        n795 = case shown="True" w1162 {
          selector: w1162 -> [_ w1168]
          frame False {
          }
          frame True {
            n796 = Not(x=w1168) -> (.not. x?=w1167:bool)
            n797 = local write "CAMERA ROI MIN TEMP"(w1167) -> ()
            n798 = call "IMAGE ANALYSIS.vi"("Enum"=POST_ANALYSIS_ENUM."MINIMIZE UI") -> ()  [unwired: 9 in, 2 out]
          }
        }
      }
    }
    n799 = local read "Auto Start Test"() -> (w915:bool)
    n800 = case shown="True" "sign in temp" {
      frame False {
      }
      frame True {
        w952 = 1 ("y")
        n801 = local read "USERNAME"() -> (w958:string)
        n802 = local read "USER ID"() -> (w955:string)
        n803 = call <vilib>:"Trim Whitespace.vi"("string"=w958) -> ("trimmed string"=w957:string)  [unwired: 1 in]
        n804 = call <vilib>:"Trim Whitespace.vi"("string"=w955) -> ("trimmed string"=w956:string)  [unwired: 1 in]
        n805 = String Length(string=w957) -> (length=w954:i32)
        n806 = String Length(string=w956) -> (length=w953:i32)
        n807 = Greater?(x=w954, y=w952) -> (0:w951:bool)
        n808 = Greater?(x=w953, y=w952) -> (0:w950:bool)
        n809 = And(x=w951, y=w950) -> (x .and. y?=w949:bool)
        n810 = case shown="True" w949 {
          frame False {
            n811 = property on="Sign In" class="Bool (strict)"("DisabledEnum"=T16."Disabled" ("Disabled")) -> ()  [unwired: 2 in, 2 out]
          }
          frame True {
            n812 = property on="Sign In" class="Bool (strict)"("DisabledEnum"=T16."Enabled" ("Disabled")) -> ()  [unwired: 2 in, 2 out]
          }
        }
      }
    }
    n813 = local read "Air Temperature"() -> (w932:bool)
    n814 = local read "Coefficient Of Friction"() -> (w933:bool)
    n815 = case shown="False" w915 {
      frame False {
        n816 = local read "Auto stop temp"() -> (w946:bool)
        n817 = case shown="True" w946 {
          frame False {
          }
          frame True {
            n818 = local write "Auto Start Temp"(FALSE ("Auto Start Temp")) -> ()
          }
        }
      }
      frame True {
        "Auto stop temp" <- TRUE ("Auto stop temp")
      }
    }
    n819 = local read "Humidity"() -> (w931:bool)
    n820 = case shown="\"HOME\"" w943 {
      frame "HOME" {
        n821 = local write "main tab sub"(enum32{"Page 1", "Page 2"}."Page 1" ("main tab sub")) -> ()
      }
      frame Default {
        n822 = local write "main tab sub"(enum32{"Page 1", "Page 2"}."Page 2" ("main tab sub")) -> ()
      }
    }
    n823 = case shown="True" w942 {
      selector: w942 -> [_ w1276]
      frame False {
      }
      frame True {
        n824 = Not(x=w1276) -> (.not. x?=w1275:bool)
        n825 = local write "Sign In"(w1275) -> ()
        n826 = local write "Main Dashboard Buttons"(T1."Test Setup" ("Main Dashboard Buttons")) -> ()
      }
    }
    n827 = case shown="\"Numeric Display\", Default" "Num/Graph" {
      frame "Numeric Display", Default {
        n828 = property on="Single/Multiple" class="RadioBtnsControl (strict)"("Visible"=FALSE) -> ()  [unwired: 2 in, 2 out]
        n829 = property on="Single - Graph" class="Ring (strict)"("Visible"=FALSE) -> ()  [unwired: 2 in, 2 out]
        n830 = local write "Main Tab Display"(T4."Dashboard 1" ("Main Tab Display")) -> ()
      }
      frame "Graph Display" {
        n831 = property on="Single/Multiple" class="RadioBtnsControl (strict)"("Visible"=TRUE) -> ()  [unwired: 2 in, 2 out]
        n832 = case shown="\"Multiple\"" "Single/Multiple" {
          frame "Single ", Default {
            n833 = property on="Single - Graph" class="Ring (strict)"("Visible"=TRUE) -> ()  [unwired: 2 in, 2 out]
            n834 = local write "Main Tab Display"(T4."Dashboard 3" ("Main Tab Display")) -> ()
          }
          frame "Multiple" {
            n835 = property on="Single - Graph" class="Ring (strict)"("Visible"=FALSE) -> ()  [unwired: 2 in, 2 out]
            n836 = local write "Main Tab Display"(T4."Dashboard 2" ("Main Tab Display")) -> ()
          }
        }
      }
    }
    n837 = local read "Stroke"() -> (w930:bool)
    n838 = local read "USERNAME"() -> (w936:string)
    n839 = local read "USER ID"() -> (w935:string)
    n840 = case shown="True" w933 {
      selector: w933 -> [_ w1211]
      frame False {
      }
      frame True {
        n841 = Not(x=w1211) -> (.not. x?=w1210:bool)
        n842 = local write "Coefficient Of Friction"(w1210) -> ()
        n843 = local write "Tab Control 2"(T6."Coefficient Of Friction" ("Tab Control 2")) -> ()
      }
    }
    n844 = case shown="True" w932 {
      selector: w932 -> [_ w1208]
      frame False {
      }
      frame True {
        n845 = Not(x=w1208) -> (.not. x?=w1206:bool)
        n846 = local write "Air Temperature"(w1206) -> ()
        n847 = local write "Tab Control 2"(T6."Air Temperature" ("Tab Control 2")) -> ()
      }
    }
    n848 = local write "Operator ID"(w935) -> ()
    n849 = case shown="True" w930 {
      selector: w930 -> [_ w1202]
      frame False {
      }
      frame True {
        n850 = Not(x=w1202) -> (.not. x?=w1200:bool)
        n851 = local write "Stroke"(w1200) -> ()
        n852 = local write "Tab Control 2"(T6."Stroke" ("Tab Control 2")) -> ()
      }
    }
    n853 = local write "tested by"(w936) -> ()
    n854 = case shown="True" w931 {
      selector: w931 -> [_ w1205]
      frame False {
      }
      frame True {
        n855 = Not(x=w1205) -> (.not. x?=w1203:bool)
        n856 = local write "Humidity"(w1203) -> ()
        n857 = local write "Tab Control 2"(T6."Humidity" ("Tab Control 2")) -> ()
      }
    }
    n858 = case shown="\"Advance\"" "Main Dashboard Buttons" {
      tunnel: [T2."HOME" ("Main Tab") T2."Test Setup" ("Main Tab") T2."Acquire" ("Main Tab") T2."Adv Scar" ("Main Tab") T2."Adv Scar Report" ("Main Tab") T2."Compare Files" ("Main Tab") T2."About" ("Main Tab") T2."Advance" ("Main Tab")] -> w940
      frame "Home", Default {
      }
      frame "Test Setup" {
      }
      frame "Dashboard" {
      }
      frame "Imaging" {
      }
      frame "Report" {
      }
      frame "Analysis" {
      }
      frame "About" {
      }
      frame "Advance" {
      }
    }
    n859 = Wait (ms)(milliseconds to wait=u32 100) -> ()  [unwired: 1 out]
    n860 = local read "Main Tab Display"() -> (w934:T4)
    n861 = local write "Main Tab"(w940) -> ()
    n862 = case shown="\"Dashboard 3\"" w934 {
      frame "Dashboard 1", Default {
        n863 = property on="Reset Graph" class="Bool (strict)"("Visible"=FALSE) -> ()  [unwired: 2 in, 2 out]
      }
      frame "Dashboard 2" {
        n864 = property on="Reset Graph" class="Bool (strict)"("Visible"=TRUE) -> ()  [unwired: 2 in, 2 out]
      }
      frame "Dashboard 3" {
        n865 = property on="Reset Graph" class="Bool (strict)"("Visible"=TRUE) -> ()  [unwired: 2 in, 2 out]
      }
    }
    n866 = local read "SCAR MEASURMENT"() -> (w922:enum32{"Auto Scar", "Manual Scar"})
    n867 = local read "Humidity"() -> (w937:bool)
    n868 = local read "Cap Live Image"() -> (w919:bool)
    n869 = local read "Sample Temperature"() -> (w929:bool)
    n870 = local read "Air Temp vs Humidity"() -> (w927:bool)
    n871 = local read "Frequency"() -> (w928:bool)
    n872 = case shown="False" w937 {
      frame False {
        n873 = local write "Humidity On Command"(TRUE ("Humidity On Command")) -> ()
        n874 = case shown="True" "Humidity Off Command" {
          selector: "Humidity Off Command" -> [_ w1218]
          frame False {
          }
          frame True {
            n875 = stacked-sequence {
              frame #0 {
                n876 = local read "WriteHumidity"() -> (w1220:string[])
                n877 = Insert Into Array(array=w1220, new element="R;1" ("new element/subarray")) -> (w1221:string[])  [unwired: 1 in]
                n878 = local write "WriteHumidity"(w1221) -> ()
              }
              frame #1 {
                n879 = Wait (ms)(milliseconds to wait=u32 2000) -> ()  [unwired: 1 out]
              }
              frame #2 {
                n880 = local read "EVENT LOG"() -> (w1227:string)
                n881 = local read "WriteHumidity"() -> (w1224:string[])
                n882 = call "Event Log.vi"("Content"="Humidity Control Off" ("string"), "EVENT LOG"=w1227) -> ("EVENT LOG"=w1228:string)  [unwired: 8 in, 1 out]
                n883 = local write "EVENT LOG"(w1228) -> ()
                n884 = Insert Into Array(array=w1224, new element="R;1" ("new element/subarray")) -> (w1225:string[])  [unwired: 1 in]
                n885 = local write "WriteHumidity"(w1225) -> ()
              }
            }
            n886 = Not(x=w1218) -> (.not. x?=w1217:bool)
            n887 = local write "Humidity Off Command"(w1217) -> ()
          }
        }
      }
      frame True {
        n888 = local write "Humidity Off Command"(TRUE ("Humidity Off Command")) -> ()
        n889 = case shown="False" "Humidity On Command" {
          selector: "Humidity On Command" -> [_ w1232]
          frame False {
          }
          frame True {
            n890 = stacked-sequence {
              frame #0 {
                n891 = local read "Set Rh"() -> (w1238:dbl)
                n892 = Number To Fractional String(number=w1238, precision (6)=i16 2) -> (F-format string=w1239:string)  [unwired: 2 in]
                n893 = local read "WriteHumidity"() -> (w1236:string[])
                n894 = Concatenate Strings("M;" ("new element/subarray"), w1239) -> (w1237:string)
                n895 = Insert Into Array(array=w1236, new element=w1237) -> (w1235:string[])  [unwired: 1 in]
                n896 = local write "WriteHumidity"(w1235) -> ()
              }
              frame #1 {
                n897 = Wait (ms)(milliseconds to wait=u32 1500) -> ()  [unwired: 1 out]
              }
              frame #2 {
                (unwired) "% RH" ("string")
                (unwired) i16 2 ("precision (6)")
                (unwired) "M;" ("new element/subarray")
                n898 = local read "Set Rh"() -> (w1246:dbl)
                n899 = Number To Fractional String(number=w1246, precision (6)=i16 2) -> (F-format string=w1243:string)  [unwired: 2 in]
                n900 = local read "WriteHumidity"() -> (w1248:string[])
                n901 = Concatenate Strings("M;" ("new element/subarray"), w1243) -> (w1247:string)
                n902 = Concatenate Strings("Humidity Set to : " ("string"), w1243, "% RH" ("string")) -> (w1241:string)
                n903 = Insert Into Array(array=w1248, new element=w1247) -> (w1249:string[])  [unwired: 1 in]
                n904 = disable-structure shown="Enabled" {
                  frame Enabled {
                    n905 = local read "EVENT LOG"() -> (w1252:string)
                    n906 = call "Event Log.vi"("Content"="Humidity Control On", "EVENT LOG"=w1252) -> ("EVENT LOG"=w1253:string)  [unwired: 8 in, 1 out]
                    n907 = local write "EVENT LOG"(w1253) -> ()
                  }
                  frame Disabled {
                  }
                }
                n908 = disable-structure shown="Enabled" {
                  disable-tunnel: w1241 -> [_ _]
                  frame Enabled {
                    n909 = local read "EVENT LOG"() -> (w1255:string)
                    n910 = call "Event Log.vi"("Content"="Humidity Control On", "EVENT LOG"=w1255) -> ("EVENT LOG"=w1256:string)  [unwired: 8 in, 1 out]
                    n911 = local write "EVENT LOG"(w1256) -> ()
                  }
                  frame Disabled {
                  }
                }
                n912 = local write "WriteHumidity"(w1249) -> ()
              }
            }
            n913 = Not(x=w1232) -> (.not. x?=w1231:bool)
            n914 = local write "Humidity On Command"(w1231) -> ()
          }
        }
      }
    }
    n915 = Equal?(x=w922, y=enum32{"Auto Scar", "Manual Scar"}."Auto Scar" ("SCAR MEASURMENT")) -> (x = y?=w918:bool)
    n916 = local read "TEST STANDARD"() -> (w925:T3)
    n917 = And(x=w919, y=w918) -> (x .and. y?=w920:bool)
    n918 = case shown="True" w920 {
      selector: w920 -> [_ w1019]
      tunnel: errorcluster {"status"=FALSE, "code"=0, "source"=""} ("error in (no error) 3") -> [_ w1020]
      frame False {
      }
      frame True {
        n919 = stacked-sequence {
          tunnel: w1020 -> [_ _ _ _ _ _ _ w1068]
          tunnel: w1019 -> [_ _ _ _ _ w1049 _ _]
          frame #0 {
            n920 = call "CAMERA LIVE FEED FGV.vi"("Enum - Menu"=CAMERA_LIVE_FEED_ENUM."CAMERA MINIMIZE") -> ()  [unwired: 9 in, 2 out]
          }
          frame #1 {
            n921 = property on="Auto Scar Check  2" class="Clust (strict)"("Visible"=TRUE) -> ()  [unwired: 2 in, 2 out]
          }
          frame #2 {
            n922 = String To Path(string="C:\\LAB-IQ\\Image Calibrate v01.dcf") -> (path=w1025:path)
            n923 = Open/Create/Replace File ("Open File")(file path (use dialog)=w1025) -> (refnum out=w1026:refnum<file>)  [unwired: 5 in, 2 out]
            n924 = for {
              N: 4 -> [_]
              tunnel: w1026 -> [w1032]
              i -> [w1028]
              n925 = Read from Text File ("Read File")(file (use dialog)=w1032) -> (text=w1033:string)  [unwired: 3 in, 3 out]
              n926 = String Subset(string=w1033, offset (0)=6, length (rest)=10 ("length (rest)")) -> (substring=w1029:string)
              n927 = Fract/Exp String To Number(string=w1029) -> (number=w1027:dbl)  [unwired: 3 in, 1 out]
              n928 = case shown="0" w1028 {
                tunnel: w1027 -> [w1034 w1035 _ w1036 _]
                frame 0 {
                  "5x Gain" <- w1034
                }
                frame 1 {
                  "10x Gain" <- w1035
                }
                frame 2 {
                }
                frame 3 {
                  "100x gain" <- w1036
                }
                frame 4, Default {
                }
              }
            }
          }
          frame #3 {
            n929 = local read "FILE 3"() -> (w1042:string)
            n930 = call <vilib>:"Trim Whitespace.vi"("string"="C:\\LAB-IQ\\images\\") -> ("trimmed string"=w1044:string)  [unwired: 1 in]
            n931 = String To Path(string=w1044) -> (path=w1043:path)
            n932 = Concatenate Strings(w1042, ".png" ("string")) -> (w1041:string)
            n933 = Build Path(base path=w1043, name or relative path=w1041) -> (appended path=w1039:path)
            "Image path" <- w1039
            n934 = Path To String(path=w1039) -> (string=w1038:string)
            n935 = call "CAMERA LIVE FEED FGV.vi"("Enum - Menu"=CAMERA_LIVE_FEED_ENUM."CAMERA SAVE", "Image Path"=w1038) -> ()  [unwired: 8 in, 2 out]
          }
          frame #4 {
            n936 = One Button Dialog(message="Image saved successfully") -> ()  [unwired: 1 in, 1 out]
          }
          frame #5 {
            n937 = local read "TEST STANDARD"() -> (w1048:T3)
            n938 = local read "Magnification len live scar"() -> (w1060:string)
            n939 = Not(x=w1049) -> (.not. x?=w1050:bool)
            n940 = local write "Cap Live Image"(w1050) -> ()
            n941 = case shown="\"ISO 12156\"" w1048 {
              tunnel: ["ASTM D6079" "ISO 12156"] -> w1047
              frame "ASTM D6079", Default {
              }
              frame "ISO 12156" {
              }
            }
            n942 = case shown="\"5x\", Default" w1060 {
              tunnel: [w1063 w1064] -> w1059
              frame "5x", Default {
                n943 = local read "5x Gain"() -> (w1063:dbl)
              }
              frame "10x" {
                # "5x"
                n944 = local read "10x Gain"() -> (w1064:dbl)
              }
            }
            n945 = local read "Image path"() -> (w1058:path)
            n946 = local read "FILE 3"() -> (w1051:string)
            n947 = call "EDGE DETCTION.vi"("GAIN VALUE"=w1059, "Image Path"=w1058) -> ("error out"=w1057:errorcluster, "return value"=w1056:cluster{string, string, dbl, dbl, dbl})  [unwired: 8 in]
            n948 = Bundle By Name(cluster=T21 {"File Name"="", "Test Method"="", "Operator"="", "Fuel Description"="", "Date and time"=""} ("Main Ref"), "File Name"=w1051, "Test Method"=w1047) -> (w1052:T21)
            n949 = call "duf file read.vi"("error in (no error)"=w1057, "Main Ref"=w1052) -> ("error out"=w1055:errorcluster, "Main Ref 2"=w1053:T21)  [unwired: 8 in]
            n950 = call "EDGE DETECTION REPORT.vi"("error in (no error)"=w1055, "return value 2"=w1056, "Main Ref"=w1053) -> ()  [unwired: 8 in, 1 out]
          }
          frame #6 {
            n951 = property on="Auto Scar Check  2" class="Clust (strict)"("Visible"=FALSE) -> ()  [unwired: 2 in, 2 out]
          }
          frame #7 {
            n952 = call "CAMERA LIVE FEED FGV.vi"("Enum - Menu"=CAMERA_LIVE_FEED_ENUM."CAMERA MINIMIZE", "error in (no error)"=w1068) -> ()  [unwired: 8 in, 2 out]
            n953 = local write "Main Dashboard Buttons"(T1."Home" ("Main Dashboard Buttons")) -> ()
            n954 = local write "Main Tab"(T2."HOME" ("Main Tab")) -> ()
          }
        }
      }
    }
    n955 = local read "Heater Button"() -> (w926:bool)
    n956 = case shown="True" w928 {
      selector: w928 -> [_ w1196]
      frame False {
      }
      frame True {
        n957 = Not(x=w1196) -> (.not. x?=w1194:bool)
        n958 = local write "Frequency"(w1194) -> ()
        n959 = local write "Tab Control 2"(T6."Frequency" ("Tab Control 2")) -> ()
      }
    }
    n960 = case shown="True" w927 {
      selector: w927 -> [_ w1193]
      frame False {
      }
      frame True {
        n961 = Not(x=w1193) -> (.not. x?=w1191:bool)
        n962 = local write "Air Temp vs Humidity"(w1191) -> ()
        n963 = local write "Tab Control 2"(T6."Air Temp vs Rh" ("Tab Control 2")) -> ()
      }
    }
    n964 = case shown="True" w929 {
      selector: w929 -> [_ w1199]
      frame False {
      }
      frame True {
        n965 = Not(x=w1199) -> (.not. x?=w1197:bool)
        n966 = local write "Sample Temperature"(w1197) -> ()
        n967 = local write "Tab Control 2"(T6."Sample Temperature" ("Tab Control 2")) -> ()
      }
    }
    n968 = case shown="\"Custom\"" w925 {
      frame "ASTM D6079", Default {
        w1172 = "ASTM D6079 TEST CONDITIONS" ("Standard 2")
        n969 = local write "Standard 2"(w1172) -> ()
        n970 = local write "Standard"(w1172) -> ()
      }
      frame "ISO 12156" {
        w1173 = "ISO 12156 TEST CONDITIONS" ("Standard 2")
        n971 = local write "Standard 2"(w1173) -> ()
        n972 = local write "Standard"(w1173) -> ()
      }
      frame "CEC F-096-A-06" {
        w1174 = "CEC F-096-A-06 TEST CONDITIONS" ("Standard 2")
        n973 = local write "Standard 2"(w1174) -> ()
        n974 = local write "Standard"(w1174) -> ()
      }
      frame "Custom" {
        w1175 = "CUSTOM TEST CONDITIONS" ("Standard 2")
        n975 = local write "Standard 2"(w1175) -> ()
        n976 = local write "Standard"(w1175) -> ()
      }
    }
    n977 = case shown="True" w926 {
      frame False {
        n978 = local write "Temperature On Command"(TRUE ("Temperature On Command")) -> ()
        n979 = case shown="True" "Temperature Off Command" {
          selector: "Temperature Off Command" -> [_ w1179]
          frame False {
          }
          frame True {
            n980 = Not(x=w1179) -> (.not. x?=w1178:bool)
            n981 = local read "EVENT LOG"() -> (w1182:string)
            n982 = local write "Temperature Off Command"(w1178) -> ()
            n983 = call "Event Log.vi"("Content"="Heater Off", "EVENT LOG"=w1182) -> ("EVENT LOG"=w1181:string)  [unwired: 8 in, 1 out]
            n984 = local write "EVENT LOG"(w1181) -> ()
          }
        }
      }
      frame True {
        n985 = local write "Temperature Off Command"(TRUE ("Temperature Off Command")) -> ()
        n986 = case shown="True" "Temperature On Command" {
          selector: "Temperature On Command" -> [_ w1186]
          frame False {
          }
          frame True {
            n987 = Not(x=w1186) -> (.not. x?=w1185:bool)
            n988 = local write "Temperature On Command"(w1185) -> ()
            n989 = disable-structure shown="Enabled" {
              disable-tunnel: "Heater On" -> [w1188 _]
              frame Enabled {
                n990 = local read "EVENT LOG"() -> (w1189:string)
                n991 = call "Event Log.vi"("Content"=w1188, "EVENT LOG"=w1189) -> ("EVENT LOG"=w1190:string)  [unwired: 8 in, 1 out]
                n992 = local write "EVENT LOG"(w1190) -> ()
              }
              frame Disabled {
              }
            }
          }
        }
      }
    }
    n993 = local read "Main Tab"() -> (w917:T2)
    n994 = case shown="\"About\"" w917 {
      frame "HOME", Default {
        w963 = T16."Enabled" ("Disabled")
        n995 = local read "Service Password enable"() -> (w962:bool)
        n996 = property on="Imaging" class="Bool (strict)"("DisabledEnum"=w963) -> ()  [unwired: 2 in, 2 out]
        n997 = property on="Dashboard" class="Bool (strict)"("DisabledEnum"=w963) -> ()  [unwired: 2 in, 2 out]
        n998 = property on="Test Setup" class="Bool (strict)"("DisabledEnum"=w963) -> ()  [unwired: 2 in, 2 out]
        n999 = property on="Analysis" class="Bool (strict)"("DisabledEnum"=w963) -> ()  [unwired: 2 in, 2 out]
        n1000 = property on="Home" class="Bool (strict)"("DisabledEnum"=w963) -> ()  [unwired: 2 in, 2 out]
        n1001 = property on="Report" class="Bool (strict)"("DisabledEnum"=w963) -> ()  [unwired: 2 in, 2 out]
        n1002 = property on="Main Dashboard Buttons" class="RadioBtnsControl (strict)"("DisabledEnum"=w963) -> ()  [unwired: 2 in, 2 out]
        n1003 = case shown="True" w962 {
          tunnel: [T16."Disabled" ("Disabled") T16."Enabled" ("Disabled")] -> w961
          frame False {
          }
          frame True {
          }
        }
        n1004 = property on="About" class="Bool (strict)"("DisabledEnum"=w961) -> ()  [unwired: 2 in, 2 out]
      }
      frame "Test Setup" {
        w968 = T16."Enabled" ("Disabled")
        n1005 = local read "Service Password enable"() -> (w967:bool)
        n1006 = property on="Dashboard" class="Bool (strict)"("DisabledEnum"=T16."Disabled" ("Disabled")) -> ()  [unwired: 2 in, 2 out]
